vi "Run.vi"(8 "error in (no error)":errorcluster caption="entrée d'erreur (pas d'erreur)", 9 "Y":string[][](array[string]), 10 "X":string[][](array[string]), 11 "Pairwise_distances_chunked.lvclass":refnum<class "Pairwise_distances_chunked.lvclass">) -> (0 "error out":errorcluster caption="sortie d'erreur", 2 "Data":T1, 3 "Pairwise_distances_chunked.lvclass":refnum<class "Pairwise_distances_chunked.lvclass">)   [LabVIEW 2020, in "Pairwise_distances_chunked.lvclass"]
doc: "Returns :\n\n- D_chunk : array or sparse matrix\nA contiguous slice of distance matrix"
uses:
  Pairwise_distances_chunked.lvclass
  Pairwise_distances_chunked.lvclass/Pairwise_distances_chunked.ctl
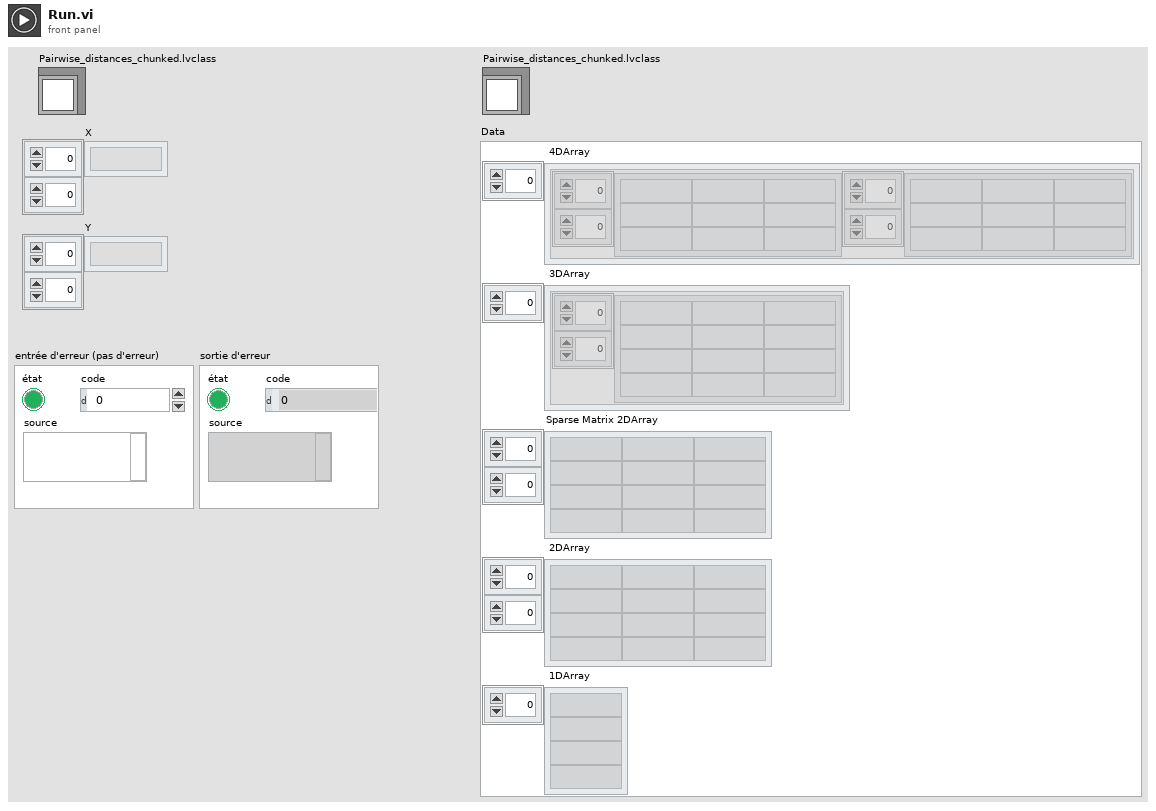
[diagram p1: front panel]
types:
  T1 = cluster{" 4DArray":cluster{"1":string[][], "2":string[][]}[], " 3DArray":cluster{"Tableau":string[][]}[], "Sparse Matrix 2DArray":string[][], " 2DArray":string[][], " 1DArray":string[]}
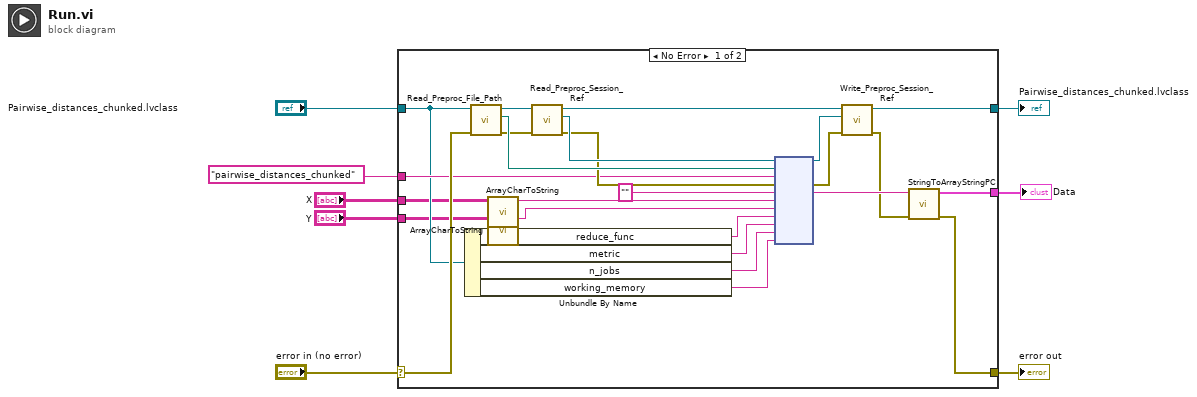
[diagram p0: block diagram]
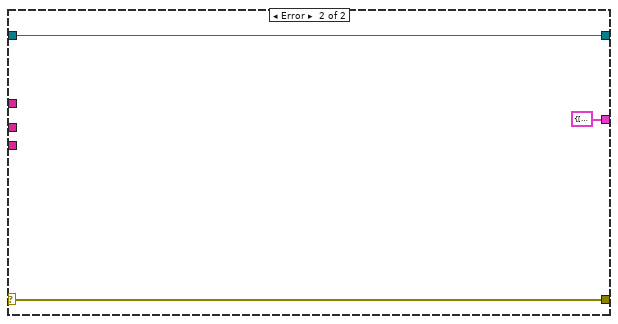
[diagram p2: hidden frame]
diagram:
  n1 = case shown="No Error" "error in (no error)" {
    selector: "error in (no error)" -> [w24 w36]
    tunnel: [w10 w36] -> w7
    tunnel: [w13 w35] -> w5
    tunnel: "Pairwise_distances_chunked.lvclass" -> [w22 w35]
    tunnel: "pairwise_distances_chunked" ("Fonction") -> [w23 _]
    tunnel: "X" -> [w17 _]
    tunnel: "Y" -> [w16 _]
    tunnel: [w9 T1 {" 4DArray"=[], " 3DArray"=[], "Sparse Matrix 2DArray"=[], " 2DArray"=[], " 1DArray"=[]} ("Data")] -> w1
    frame No Error {
      n2 = Unbundle By Name(w22) -> ("reduce_func"=w21:string, "metric"=w20:string, "n_jobs"=w19:string, "working_memory"=w18:string)
      n3 = call-dynamic "Read_Preproc_File_Path.vi"("error in (no error)"=w24, "Python in"=w22) -> ("error out"=w28:errorcluster, "File_Path"=w31:path, "Python out"=w33:refnum<class "Pairwise_distances_chunked.lvclass">)  [unwired: 7 in]
      n4 = call "ArrayCharToString.vi"("TAB"=w17) -> ("Instruction"=w15:string)  [unwired: 10 in]
      n5 = call "ArrayCharToString.vi"("TAB"=w16) -> ("Instruction"=w14:string)  [unwired: 10 in]
      n6 = call-dynamic "Read_Preproc_Session_Ref.vi"("error in (no error)"=w28, "Python in"=w33) -> ("error out"=w29:errorcluster, "Session_ref"=w30:refnum<k35>, "Python out"=w32:refnum<class "Pairwise_distances_chunked.lvclass">)  [unwired: 7 in]
      n7 = node(w30, w31, w23, w29, "", w15, w14, w21, w20, w19, w18) -> (w25:refnum<k35>, w27:errorcluster, w12:string)  [unwired: 6 in, 2 out]
      n8 = call-dynamic "Write_Preproc_Session_Ref.vi"("error in (no error)"=w27, "Session_ref"=w25, "Python in"=w32) -> ("error out"=w11:errorcluster, "Python out"=w13:refnum<class "Pairwise_distances_chunked.lvclass">)  [unwired: 7 in]
      n9 = call "StringToArrayStringPC.vi"("sortie d'erreur"=w11, "Return value"=w12) -> ("sortie d'erreur"=w10:errorcluster, "Data"=w9:T1)  [unwired: 8 in]
    }
    frame Error {
    }
  }
  "error out" <- w7
  "Pairwise_distances_chunked.lvclass" <- w5
  "Data" <- w1
